vi "Run.vi"(6 "clone#":i32, 11 "target in":refnum<class "Base Target.lvclass">) -> (3 "target out":refnum<class "Base Target.lvclass">)   [LabVIEW 2020, in "NI_TargetHelper.lvlib" / "Base Target.lvclass"]
uses:
  <vilib>/TargetSupport/NI_TargetHelper/Base Target/Base Target.lvclass
panel:
  in  "done":bool
  in  "abort":bool
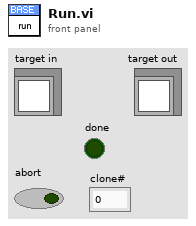
[diagram p1: front panel]
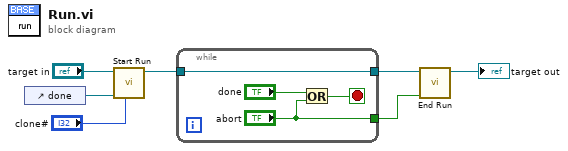
[diagram p0: block diagram]
diagram:
  n1 = control-ref of="done"() -> (w6:refnum<vi>)
  n2 = call-dynamic "Start Run.vi"("clone#"="clone#", "done ref"=w6, "target in"="target in") -> ("target out"=w5:refnum<class "Base Target.lvclass">)  [unwired: 8 in]
  n3 = while {
    tunnel: [w11] -> w3
    tunnel: w5 -> [w11]
    tunnel: ["abort"] -> w2
    stop <- w9 stop-if-true
    n4 = Or(x="done", y="abort") -> (x .or. y?=w9:bool)
  }
  n5 = call-dynamic "End Run.vi"("abort"=w2, "target in"=w3) -> ("target out"=→"target out":refnum<class "Base Target.lvclass">)  [unwired: 9 in]
